vi "x502_open.vi"(2 "error out 2":errorcluster, 3 "serial":string) -> (0 "error out":errorcluster, 1 "x502 out":refnum<k24>)   [LabVIEW 2018]
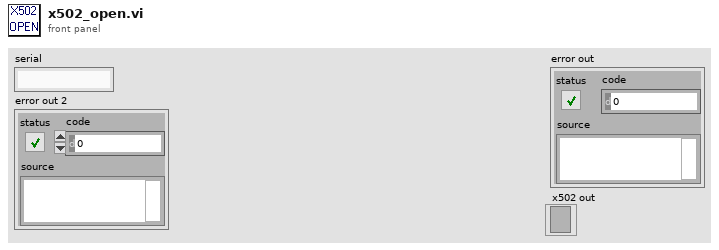
[diagram p1: front panel]
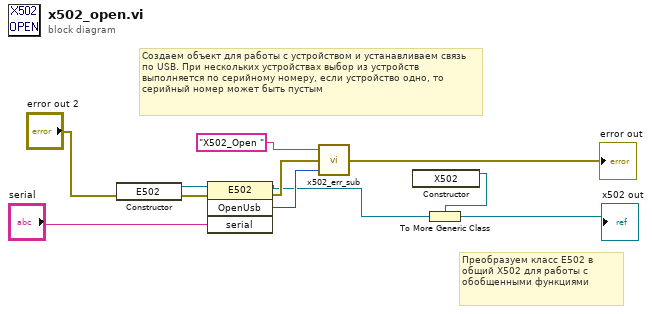
[diagram p0: block diagram]
diagram:
  # "Преобразуем класс E502 в общий X502 для работы с обобщенными функциями"
  # "Создаем объект для работы с устройством и устанавливаем связь по USB. При нескольких устройствах выбор из устройств выполняется по серийному номеру, если устройство одно, то серийный номер может быть пустым"
  n1 = constructor class="E502"(error in="error out 2") -> (reference out=w8:refnum<k24>, error out=w7:errorcluster)  [unwired: 2 in, 1 out]
  n2 = invoke class="E502" method="OpenUsb"(reference=w8, error in=w7, "serial"="serial") -> (reference out=w5:refnum<k24>, error out=w10:errorcluster, "OpenUsb"=w11:i32)  [unwired: 1 in, 1 out]
  n3 = call "x502_err_sub.vi"("Error code"=w11, "error in (no error)"=w10, "Error descr"="X502_Open ") -> ("error out"=→"error out":errorcluster)
  n4 = constructor class="X502"() -> (reference out=w6:refnum<k24>)  [unwired: 3 in, 2 out]
  n5 = To More Generic Class(target class=w6, reference=w5) -> (generic class reference=→"x502 out":refnum<k24>)
